vi "integrated_prac.vi"() -> ()   [LabVIEW 2014]
uses:
  <vilib>/Motion/FlexMotion/CustomControls/CustomControls.llb/AxisOrVectorSpace To Configure.flx
  <vilib>/Motion/FlexMotion/FunctionsVIs/StartStopMotion.llb/Start Motion (8 axes).flx
  <vilib>/Motion/FlexMotion/FunctionsVIs/Trajectory.llb/Check Move Complete Status (8 axes).flx
  <vilib>/Motion/FlexMotion/FunctionsVIs/StartStopMotion.llb/Stop Motion (8 axes).flx
  <instrlib>/KD Scientific 2XX Series/KD Scientific 2XX Series.lvlib
panel:
  in  "Stop Type (Decel)":enum16{"Decelerate", "Halt", "Kill"}(ring)
  in  "Velocity (10000)":i32=10000 min=-20000000 max=20000000
  in  "Target Position (0)":i32
  in  "Position Mode (Absolute)":T1(ring)
  in  "error in (no error) 2":errorcluster
  in  "Axis or Vector Space":T2=1 items=["Axis 1"=1, "Axis 2"=2, "Axis 3"=3, "Axis 4"=4, "Axis 5"=5, "Axis 6"=6, "Axis 7"=7, "Axis 8"=8, "Vector Space 1"=17, "Vector Space 2"=18, "Vector Space 3"=19, "Vector Space 4"=20]
  in  "Board ID":T3=1 min=1 max=32 step=1
  out "Units":string
  out "Delivered Volume":dbl
  in  "stop":bool
  out "Status":T4
  in  "Flow Rate (5)":dbl=5.0
  in  "Units (0: milliliters)":u16(ring) items=["milliliters (ml)", "microliters (ul)"]
  in  "Volume (100)":dbl=100.0
  in  "Diameter (8.75 mm)":dbl=8.75
  in  "Mode (infuse)":u16(ring) items=["Infuse", "Withdraw", "Infuse-Withdraw", "Withdraw-Infuse", "Continuous"]
  in  "Address (0)":i32
  in  "error in (no error)":errorcluster
  in  "Baud Rate (9600)":u32(ring)=9600 items=["300"=300, "1200"=1200, "2400"=2400, "4800"=4800, "9600"=9600]
  in  "VISA resource name":refnum<visa-resource-name>
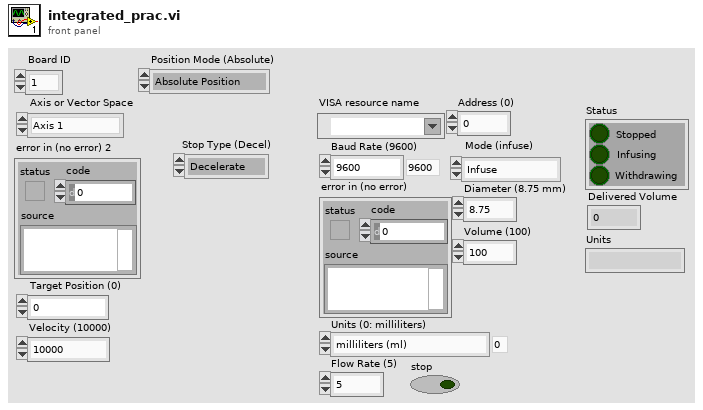
[diagram p1: front panel]
types:
  T1 = enum16{"Absolute Position", "Relative Position", "Velocity", "Relative to Cap Pos", "Modulus Position", "Absolute Contouring", "Relative Contouring"}
  T2 = typedef "AxisOrVectorSpace To Configure.flx" = u16
  T3 = typedef "Board Id" = u8
  T4 = cluster{"Stopped":bool, "Infusing":bool, "Withdrawing":bool}
  T5 = typedef "Bd Id Out" = u8
  T6 = typedef "Resource Out (Enum).flx" = u16
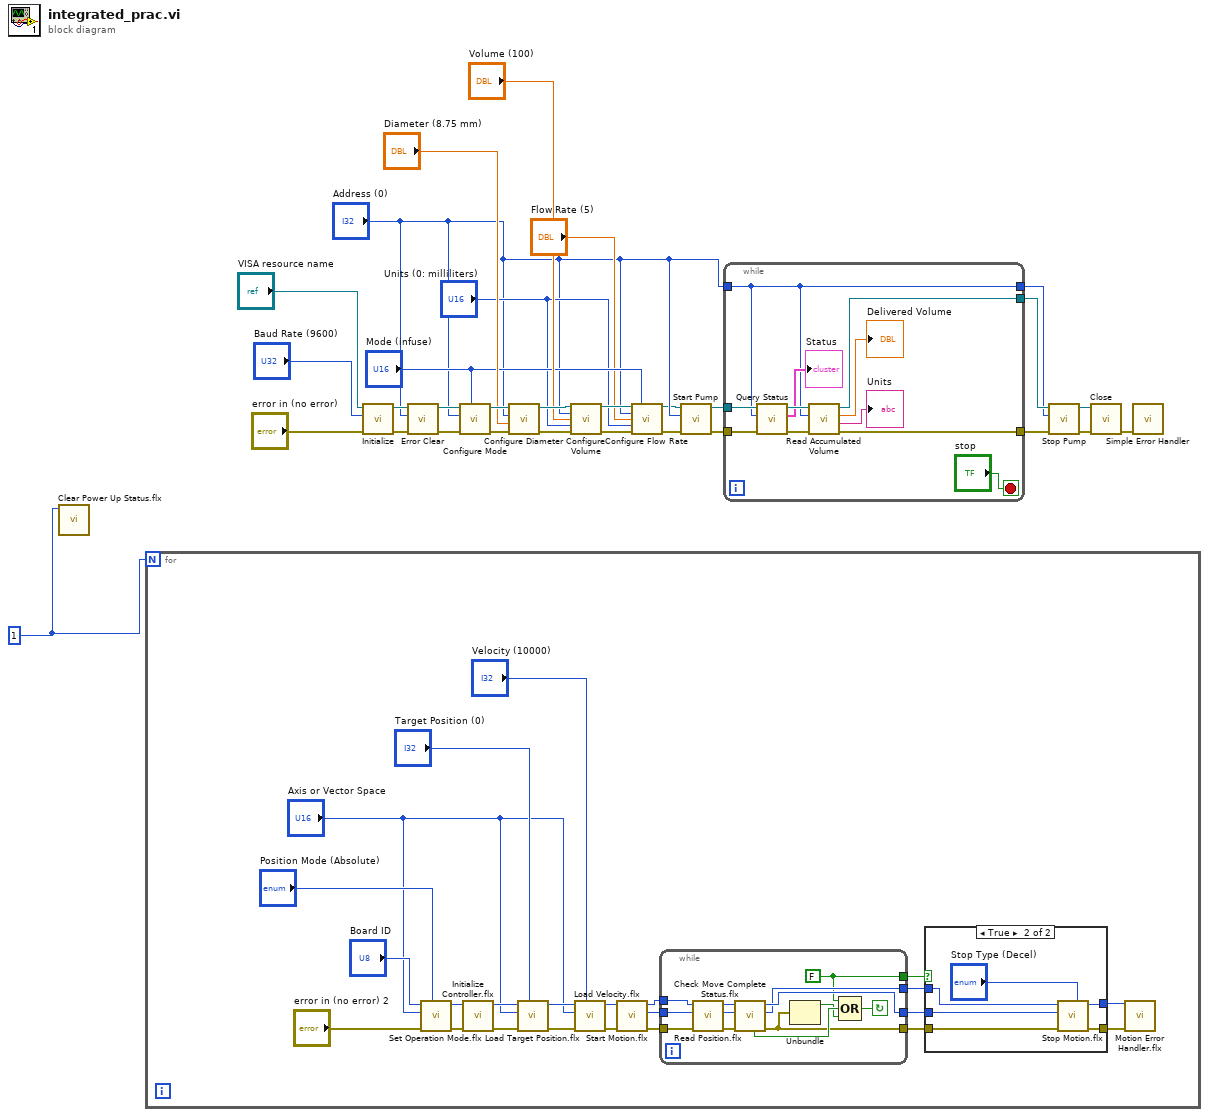
[diagram p0: block diagram]
diagram:
  w1 = T3 1 ("Board ID")
  n1 = call <vilib>:"Clear Power Up Status.flx"("Board ID"=w1) -> ()  [unwired: 6 in, 2 out]
  n2 = for {
    N: w1 -> [_]
    n3 = call <vilib>:"Set Operation Mode.flx"("Position Mode (Absolute)"="Position Mode (Absolute)", "error in (no error)"="error in (no error) 2", "Axis or Vector Space"="Axis or Vector Space", "Board ID"="Board ID") -> ("error out"=w49:errorcluster, "Bd ID Out"=w50:T5)  [unwired: 2 in, 1 out]
    n4 = call <vilib>:"Initialize Controller.flx"("error in (no error)"=w49, "Board ID"=w50) -> ("error out"=w46:errorcluster, "Bd ID Out"=w47:T5)  [unwired: 6 in]
    n5 = call <vilib>:"Load Target Position.flx"("Target Position (0)"="Target Position (0)", "error in (no error)"=w46, "Axis"="Axis or Vector Space", "Board ID"=w47) -> ("error out"=w44:errorcluster, "Bd ID Out"=w45:T5)  [unwired: 3 in, 1 out]
    n6 = call <vilib>:"Load Velocity.flx"("Velocity (10000)"="Velocity (10000)", "error in (no error)"=w44, "Axis or Vector Space"="Axis or Vector Space", "Board ID"=w45) -> ("error out"=w40:errorcluster, "Bd ID Out"=w41:T5)  [unwired: 3 in, 1 out]
    n7 = call-poly <vilib>:"Start Motion.flx"("error in (no error)"=w40, "Board ID"=w41) -> ("error out"=w37:errorcluster, "Resource Output"=w39:T6, "Bd ID Out"=w38:T5)  [unwired: 4 in]
    n8 = while {
      tunnel: w39 -> [w74]
      tunnel: w38 -> [w73]
      tunnel: w37 -> [w72]
      tunnel: [w65] -> w34
      tunnel: [w64] -> w35
      tunnel: [w63] -> w36
      tunnel: [w62] -> w33
      stop <- w66 continue-if-true
      w62 = FALSE
      n9 = call <vilib>:"Read Position.flx"("error in (no error)"=w72, "Axis"=w74, "Board ID"=w73) -> ("error out"=w70:errorcluster, "Resource Output"=w69:T6, "Bd ID Out"=w71:T5)  [unwired: 3 in, 1 out]
      n10 = call-poly <vilib>:"Check Move Complete Status.flx"("error in (no error)"=w70, "Axis or Vector Space"=w69, "Board ID"=w71) -> ("error out"=w65:errorcluster, "Resource Output"=w63:T6, "Bd ID Out"=w64:T5, "Move Complete"=w68:bool)  [unwired: 3 in]
      n11 = Unbundle(w65) -> ("status"=w67:bool)  [unwired: 2 out]
      n12 = Compound Arithmetic op=OR(w62, w68, w67) -> (w66:bool)
    }
    n13 = case shown="True" w33 {
      tunnel: w36 -> [w55 w61]
      tunnel: w35 -> [_ w60]
      tunnel: w34 -> [w54 w59]
      tunnel: [w55 w57] -> w32
      tunnel: [w54 w56] -> w31
      frame False {
      }
      frame True {
        n14 = call-poly <vilib>:"Stop Motion.flx"("Stop Type (Decel)"="Stop Type (Decel)", "error in (no error)"=w59, "Axis or Vector Space"=w60, "Board ID"=w61) -> ("error out"=w56:errorcluster, "Bd ID Out"=w57:T5)  [unwired: 3 in, 1 out]
      }
    }
    n15 = call <vilib>:"Motion Error Handler.flx"("Board ID"=w32, "error in (no error)"=w31) -> ()  [unwired: 9 in, 5 out]
  }
  n16 = call <instrlib>:"Initialize.vi"("error in (no error)"="error in (no error)", "Baud Rate (9600)"="Baud Rate (9600)", "VISA resource name"="VISA resource name") -> ("error out"=w26:errorcluster, "VISA resource name out"=w27:refnum<visa-resource-name>)  [unwired: 7 in]
  n17 = call <instrlib>:"Error Clear.vi"("error in (no error)"=w26, "Address (0)"="Address (0)", "VISA resource name"=w27) -> ("error out"=w24:errorcluster, "VISA resource name out"=w25:refnum<visa-resource-name>)  [unwired: 6 in, 1 out]
  n18 = call <instrlib>:"Configure Mode.vi"("Mode (infuse)"="Mode (infuse)", "error in (no error)"=w24, "Address (0)"="Address (0)", "VISA resource name"=w25) -> ("error out"=w14:errorcluster, "VISA resource name out"=w15:refnum<visa-resource-name>)  [unwired: 6 in]
  n19 = call <instrlib>:"Configure Diameter.vi"("error in (no error)"=w14, "Diameter (8.75 mm)"="Diameter (8.75 mm)", "Address (0)"="Address (0)", "VISA resource name"=w15) -> ("error out"=w11:errorcluster, "VISA resource name out"=w12:refnum<visa-resource-name>)  [unwired: 6 in]
  n20 = call <instrlib>:"Configure Volume.vi"("VISA resource name"=w12, "Address (0)"="Address (0)", "Volume (100)"="Volume (100)", "Units (0: milliliters)"="Units (0: milliliters)", "error in (no error)"=w11) -> ("VISA resource name out"=w9:refnum<visa-resource-name>, "error out"=w8:errorcluster)  [unwired: 9 in]
  n21 = call <instrlib>:"Configure Flow Rate.vi"("VISA resource name"=w9, "Mode (infuse)"="Mode (infuse)", "Address (0)"="Address (0)", "Flow Rate (5)"="Flow Rate (5)", "Units (0: milliliters per minute)"="Units (0: milliliters)", "error in (no error)"=w8) -> ("VISA resource name out"=w3:refnum<visa-resource-name>, "error out"=w2:errorcluster)  [unwired: 8 in]
  n22 = call <instrlib>:"Start Pump.vi"("error in (no error)"=w2, "Address (0)"="Address (0)", "VISA resource name"=w3) -> ("error out"=w22:errorcluster, "VISA resource name out"=w23:refnum<visa-resource-name>)  [unwired: 7 in]
  n23 = while {
    tunnel: w23 -> [w85]
    tunnel: w22 -> [w84]
    tunnel: "Address (0)" -> [w76]
    tunnel: [w78] -> w21
    tunnel: [w77] -> w20
    tunnel: [w76] -> w19
    stop <- "stop" stop-if-true
    n24 = call <instrlib>:"Query Status.vi"("error in (no error)"=w84, "Address (0)"=w76, "VISA resource name"=w85) -> ("error out"=w82:errorcluster, "Status"=→"Status":T4, "VISA resource name out"=w83:refnum<visa-resource-name>)  [unwired: 6 in]
    n25 = call <instrlib>:"Read Accumulated Volume.vi"("error in (no error)"=w82, "Address (0)"=w76, "VISA resource name"=w83) -> ("error out"=w77:errorcluster, "Units"=→"Units":string, "Delivered Volume"=→"Delivered Volume":dbl, "VISA resource name out"=w78:refnum<visa-resource-name>)  [unwired: 5 in]
  }
  n26 = call <instrlib>:"Stop Pump.vi"("error in (no error)"=w20, "Address (0)"=w19, "VISA resource name"=w21) -> ("error out"=w17:errorcluster, "VISA resource name out"=w18:refnum<visa-resource-name>)  [unwired: 7 in]
  n27 = call <instrlib>:"Close.vi"("error in (no error)"=w17, "VISA resource name"=w18) -> ("error out"=w16:errorcluster)  [unwired: 9 in]
  n28 = call <vilib>:"Simple Error Handler.vi"("error in (no error)"=w16) -> ()  [unwired: 4 in, 5 out]
